vi "Aipuff-Pulse.vi"(7 "Device reference":refnum<vi>, 8 "error in (no error)":errorcluster, 9 "Eventstring":string="auto-generate", 11 "Square sequence":T1=[{"Frequency (Hz)"=20.0, "Duty Cycle"=5.0, "Amplitude (V)"=5.0, "Duration (ms)"=100.0}]) -> (0 "error out":errorcluster)   [LabVIEW 2015]
doc: "Pulses a juicer valve.\n\nDevice reference: which valve?\nDuration: how long to open for?\n--positive: specifies open duration in ms\n--unwired or 0: accept default from valve ref.\n--negative: open indefinitely\nEventstring: used for timestamping\n--empty: no timestamp will be generated\n--unwired or \"auto-generate\": TS w/ default eventstring\n--otherwise: TS with user-provided string\nAcutal duration: the actual commanded pulse duration. Useful if you decided to use the default value.\n\nThe default eventstring is:\n[valve name].open.[duration]\nwhere [valve name] is the referenced valve's front panel label text and [duration] will have the actual duration filled in if the Duration input was left unwired (or set to 0)."
uses:
  Typedefs/Airpuff- Square sequence.ctl
  Typedefs/Speaker.ctl
  Rack/Typedefs/OutputRequest refnum.ctl
  Rack/Typedefs/OutputRequest.ctl
  Rack/Typedefs/InputData cluster.ctl
  Rack/Methods/Port drivers/DigitalInput-DataCluster.ctl
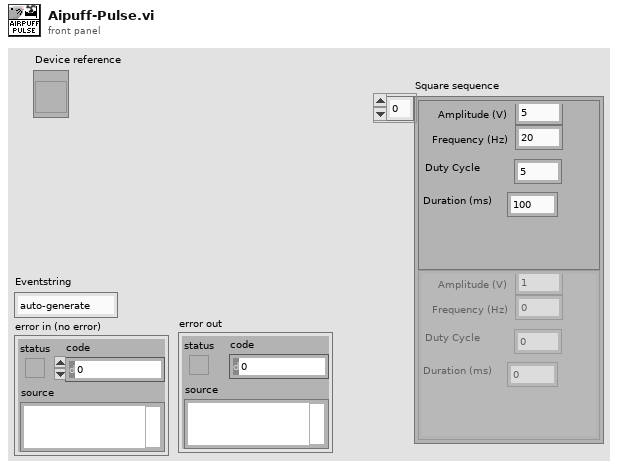
[diagram p1: front panel]
types:
  T1 = typedef "Airpuff- Square sequence.ctl" = cluster{"Frequency (Hz)":dbl, "Duty Cycle":dbl, "Amplitude (V)":dbl, "Duration (ms)":dbl}[]
  T2 = typedef "Speaker.ctl" = cluster{"Settings":cluster{"Portname":string, "Index":i32, "Timestamp portname":string}, "OutputRequest event ref":T3, "InputData reference":refnum<vi>}
  T3 = typedef "OutputRequest refnum.ctl" = refnum<user-event>
  T4 = typedef "OutputRequest.ctl" = cluster{"Target":string, "Command":string}
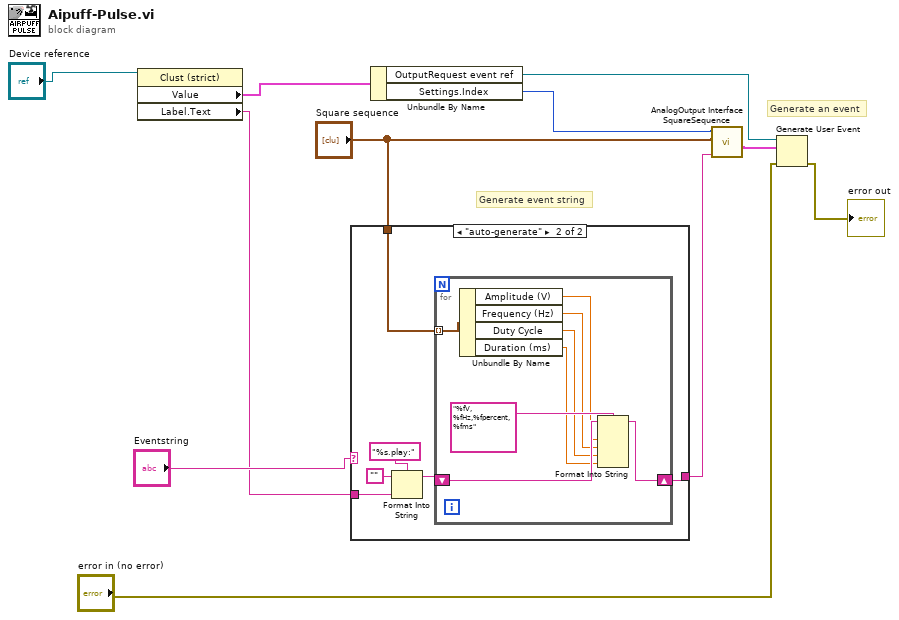
[diagram p0: block diagram]
diagram:
  # "Generate event string"
  # "Generate an event"
  n1 = property class="Clust (strict)"(reference="Device reference") -> ("Value"=w3:T2, "Label.Text"=w2:string)  [unwired: 1 in, 2 out]
  n2 = case shown="\"auto-generate\"" "Eventstring" {
    selector: "Eventstring" -> [w12 _]
    tunnel: w2 -> [_ w16]
    tunnel: [w12 w13] -> w6
    tunnel: "Square sequence" -> [_ w15]
    frame Default {
      # "Use user-provided string"
    }
    frame "auto-generate" {
      n3 = Format Into String(format string="%s.play:", initial string="", w16) -> (resulting string=w14:string)  [unwired: 1 in, 1 out]
      n4 = for {
        tunnel: w15 -> [w25] mode=indexing
        shift-right: [w23] -> w13
        shift-left: w14 -> [w24]
        n5 = Unbundle By Name(w25) -> ("Amplitude (V)"=w22:dbl, "Frequency (Hz)"=w21:dbl, "Duty Cycle"=w20:dbl, "Duration (ms)"=w19:dbl)
        n6 = Format Into String(format string="%fV, %fHz,%fpercent, %fms", initial string=w24, w22, w21, w20, w19) -> (resulting string=w23:string)  [unwired: 1 in, 1 out]
      }
    }
  }
  n7 = Unbundle By Name(w3) -> ("OutputRequest event ref"=w11:T3, "Settings.Index"=w7:i32)
  n8 = call "AnalogOutput Interface SquareSequence.vi"("Eventstring"=w6, "Square sequence"="Square sequence", "Port index"=w7) -> ("OutputRequest"=w5:T4)  [unwired: 8 in]
  n9 = Generate User Event(user event=w11, event data cluster=w5, error in="error in (no error)") -> (error out=→"error out":errorcluster)  [unwired: 1 in, 1 out]
